vi "BuildThermomechanicalStave.vi"() -> ()   [LabVIEW 2016]
doc: "This VI is the overarching framework for the ITk Stave Assembly at Brookhaven National Lab. This VI coordinates all SubVIs so that the user can execute all phases of construction: Calibration, Module Placement, and Final Survey."
uses:
  <vilib>/userdefined/High Color/IMAQdx.ctl
  C:/Users/sciollalab/Documents/Brandeis-BNL/LabVIEW_Codes/BNL_ThermomechanicalStave/AerotechLibraries/Bin/Aerotech.A3200.dll
  AerotechLibraries/Bin/Aerotech.A3200.dll
  <vilib>/Utility/file.llb/Write Delimited Spreadsheet (DBL).vi
  <vilib>/vision/driver/NI_Vision_Acquisition_Software.lvlib
panel:
  out "Current time and temperature":string[](array[string])
  out "Wait to capture [ms]":u32
  in  "Wait time [s]":dbl=3.5
  in  "N pix/um images":i32=1
  out "Inputs: Collect images":T2={"Session in"="", "Axes Speeds [mm/s]"={"X Speed"=10.0, "Y Speed"=10.0, "Z Speed"=10.0}, "XYZ .NET Refnum in"=refnum, "Current image"=refnum, "Stage position"=refnum, "Moving"=refnum}
  out "XYZ Stage Control":refnum<k24>
  out "Baseline Z [mm]":dbl
  in  "Placement tolerance [um]":dbl=10.0
  out "Module Progress Report":T3(array[cluster])
  out "Surveyed?":bool
  out "Mounted?":bool
  out "Calibrated?":bool
  in  "N Modules":i32=13
  out "Calibrated module height":dbl
  out "Calibrated stave basis [mm]":dbl[][](array[numeric])
  out "Module fiducials in the XYZ stage's basis":T4(graph)=[{"Generated List of Module Coordinates"=[0.0, 280.05, 574.05, 868.05, 1162.05], "Generated List of Module Coordinates"=[0.0, 0.0, 0.0, 0.0, 0.0]}, {"Generated List of Module Coordinates"=[-7.689999999999998, 87.79, 87.79, -7.689999999999998, 90.31, 185.79000000000002, 185.79000000000002, 90.31, 188.31, 283.79, 283.79, 188.31, 286.31, 381.79, 381.79, 286.31, 384.31, 479.79, 479.79, 384.31, 482.30999999999995, 577.79, 577.79, 482.30999999999995, 580.31, 675.79, 675.79, 580.31, 678.31, 773.79, 773.79, 678.31, 776.31, 871.79, 871.79, 776.31, 874.31, 969.79, 969.79, 874.31, 972.31, 1067.79, 1067.79, 972.31, 1070.31, 1165.79, 1165.79, 1070.31, 1168.31, 1263.79, 1263.79, 1168.31], "Generated List of Module Coordinates"=[-113.212, -113.212, -16.13199999999999, -16.13199999999999, -113.212, -113.212, -16.13199999999999, -16.13199999999999, -113.212, -113.212, -16.13199999999999, -16.13199999999999, -113.212, -113.212, -16.13199999999999, -16.13199999999999, -113.212, -113.212, -16.13199999999999, -16.13199999999999, -113.212, -113.212, -16.13199999999999, -16.13199999999999, -113.212, -113.212, -16.13199999999999, -16.13199999999999, -113.212, -113.212, -16.13199999999999, -16.13199999999999, -113.212, -113.212, -16.13199999999999, -16.13199999999999, -113.212, -113.212, -16.13199999999999, -16.13199999999999, -113.212, -113.212, -16.13199999999999, -16.13199999999999, -113.212, -113.212, -16.13199999999999, -16.13199999999999, -113.212, -113.212, -16.13199999999999, -16.13199999999999]}, {"Generated List of Module Coordinates"=[40.050000000000004, 138.05, 236.05, 334.05, 432.05, 530.05, 628.05, 726.05, 824.05, 922.05, 1020.05, 1118.05, 1216.05], "Generated List of Module Coordinates"=[-64.672, -64.672, -64.672, -64.672, -64.672, -64.672, -64.672, -64.672, -64.672, -64.672, -64.672, -64.672, -64.672]}]
  in  "Home stage?":bool
  out "Calib Pattern":T5
  out "Autofocus":T5
  out "Stave origin":T5
  in  "XYZ Stage Frame: Coordinates for calibration":T6={"Stave origin"={"X [mm]"=-628.0, "Y [mm]"=142.3, "Z [mm]"=22.0}, "Autofocus"={"X [mm]"=-597.0, "Y [mm]"=132.0, "Z [mm]"=18.0}, "Calib Pattern"={"X [mm]"=-560.0, "Y [mm]"=112.0, "Z [mm]"=13.9}}
  out "Focusing test interval [mm]":dbl
  out "Stepsize [mm]":dbl
  in  "Camera working distance scan":T7={"Stepsize [mm]"=0.2, "Focusing test interval [mm]"=1.5} {"Focusing test interval [mm]" format="%#_13g"}
  out "Calibration Results":T8 {"Camera calibration results"."Working distance to stave [mm]" format="%#_13g"}
  out "delta Z":dbl
  in  "Reports path":path=path "C:/Users/Aerotech/cernbox/BNL/Stave Assembly Records/2017-04-05"
  in  "Code path":path=path "C:/Users/Aerotech/Documents/BNL_ThermomechanicalStave"
  out "Calibrated stave origin (X,Y) [mm]":dbl[](array[numeric])
  in  "Tape Type":enum16{"Stereo", "Axial"}(ring)=enum."Axial"
  out "Angle between stave and xyz stage":dbl
  in  "Module fiducial marker":T9(ring)=enum."Mark B"
  out "Average microns/pixel":ext
  out "Optimized Z [mm]":dbl format="%#_13g"
  out "Session Out":T1="cam0"
  out "Current stage position [mm]":cluster{"X":dbl, "Y":dbl, "Z":dbl}
  out "Moving":bool
  out "Stage homed":bool
  in  "Axis Speeds":T10={"X [mm/s]"=10.0, "Y [mm/s]"=10.0, "Z [mm/s]"=10.0}
  out "Current field of view":T11(plugin-control)
  in  "Camera Name":refnum<k21>="cam1" caption="IMAQdx Session"
  in  "Program Errors":errorcluster
  out "Current Build Phase":string="Going to nominal stave origin..."
  # "BUILD THERMOMECHANICAL STAVE"
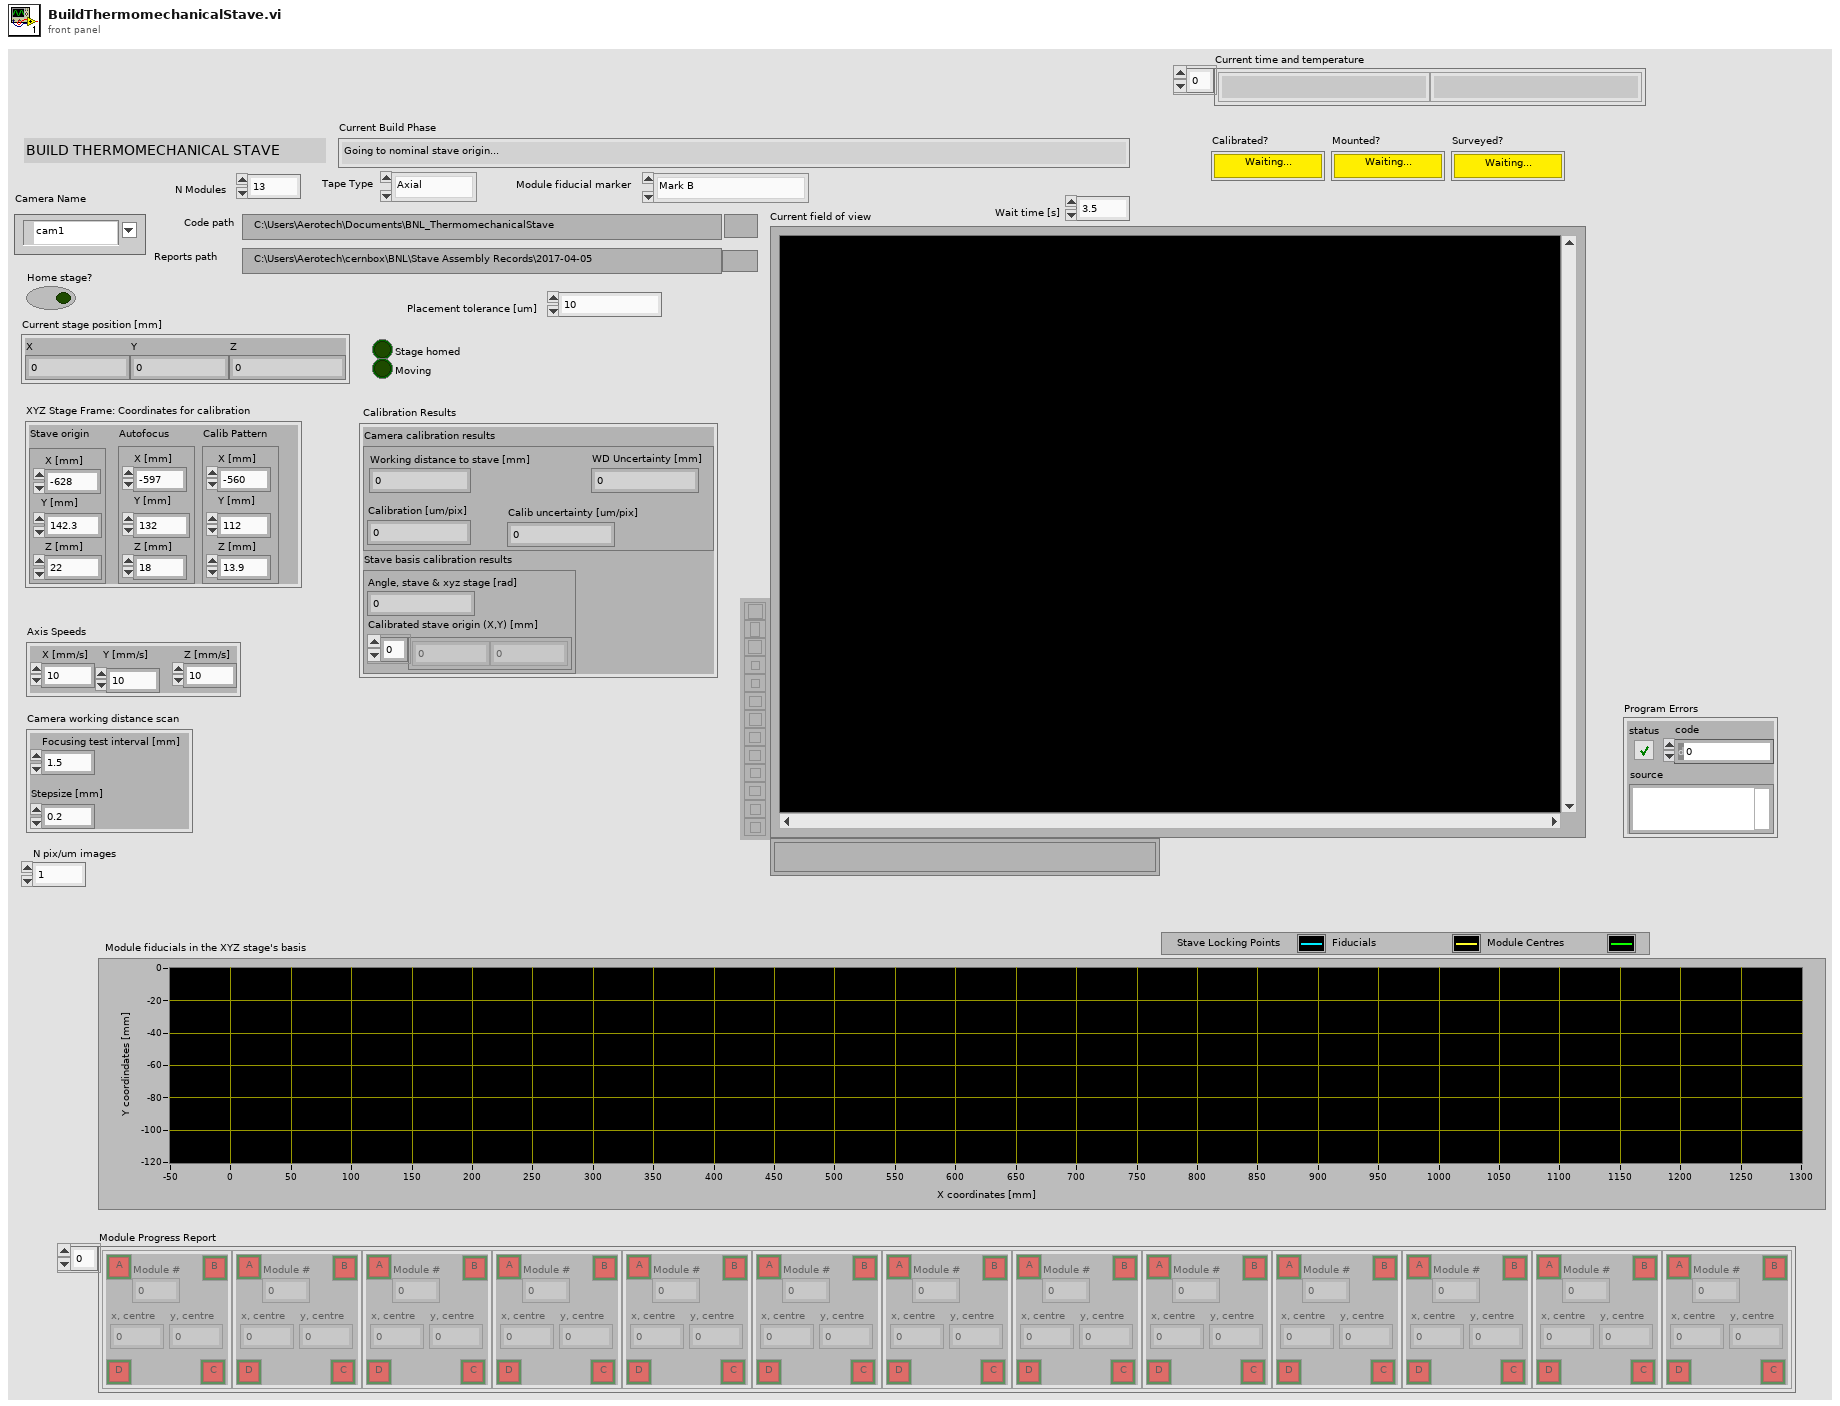
[diagram p1: front panel]
types:
  T1 = typedef "IMAQdx.ctl" = refnum<k21>
  T2 = cluster{"Session in":T1, "Axes Speeds [mm/s]":cluster{"X Speed":dbl, "Y Speed":dbl, "Z Speed":dbl}, "XYZ .NET Refnum in":refnum<k24>, "Current image":refnum<vi>, "Stage position":refnum<vi>, "Moving":refnum<vi>}
  T3 = cluster{"A":bool, "x, centre":dbl, "y, centre":dbl, "Module #":i32, "B":bool, "D":bool, "C":bool}[]
  T4 = cluster{"Generated List of Module Coordinates":dbl[], "Generated List of Module Coordinates":dbl[]}[]
  T5 = cluster{"X [mm]":dbl, "Y [mm]":dbl, "Z [mm]":dbl}
  T6 = cluster{"Stave origin":cluster{"X [mm]":dbl, "Y [mm]":dbl, "Z [mm]":dbl}, "Autofocus":cluster{"X [mm]":dbl, "Y [mm]":dbl, "Z [mm]":dbl}, "Calib Pattern":cluster{"X [mm]":dbl, "Y [mm]":dbl, "Z [mm]":dbl}}
  T7 = cluster{"Stepsize [mm]":dbl, "Focusing test interval [mm]":dbl}
  T8 = cluster{"Camera calibration results":cluster{"Calibration [um/pix]":dbl, "Working distance to stave [mm]":dbl, "Calib uncertainty [um/pix]":dbl, "WD Uncertainty [mm]":dbl}, "Stave basis calibration results":cluster{"Angle, stave & xyz stage [rad]":dbl, "Calibrated stave origin (X,Y) [mm]":dbl[]}}
  T9 = enum16{"Mark C", "Mark B", "Strip Corner", "[None]"}
  T10 = cluster{"X [mm/s]":dbl, "Y [mm/s]":dbl, "Z [mm/s]":dbl}
  T11 = typedef "IMAQ Image.ctl" = refnum<image>
  T12 = cluster{"X Position Feedback":dbl, "Y Position Feedback":dbl, "Z Position Feedback":dbl}
  T13 = cluster{"Final X":dbl, "Final Y":dbl, "Final Z":dbl}
  T14 = typedef "Image Type" = u32
  T15 = cluster{"Update X [mm]":dbl, "Update Y [mm]":dbl, "Update Z [mm]":dbl}
  T16 = cluster{"Update X [mm]":dbl, "Update Y [mm]":dbl, "Z [mm]":dbl}
  T17 = cluster{"Camera session out":T1, "Axis Speeds":cluster{"X [mm/s]":dbl, "Y [mm/s]":dbl, "Z [mm/s]":dbl}, "XYZ Stage Control":refnum<k24>, "Current field of view":refnum<vi>, "Current stage position [mm]":refnum<vi>, "Moving":refnum<vi>}
  T18 = cluster{"Session out":T1, "Captured positions":dbl[][], "XYZ .NET Refnum out":refnum<k24>}
  T19 = cluster{"Calibrated stave basis [mm]":dbl[], "Calibrated stave basis [mm]":dbl[]}
  T20 = cluster{"Calibrated stave basis [mm]":dbl[], "Calibrated stave basis [mm]":dbl[]}[]
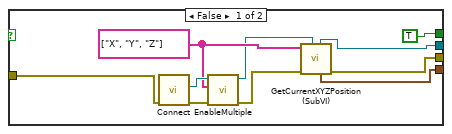
[diagram p2: hidden frame]
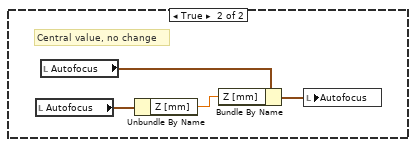
[diagram p13: hidden frame]
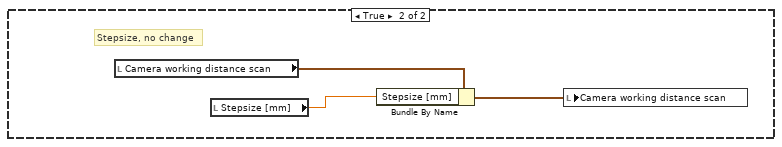
[diagram p14: hidden frame]
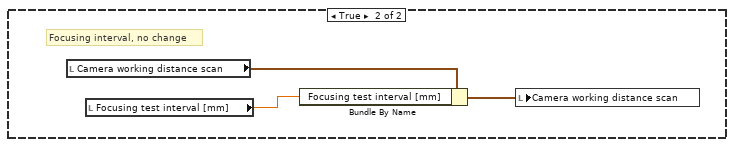
[diagram p15: hidden frame]
diagram:
  n1 = while {
    stop <- w17 stop-if-true
    # "Temperature monitoring"
    n2 = Wait (ms)(milliseconds to wait=u32 1000) -> ()  [unwired: 1 out]
    n3 = call "TimeAndTemperature (SubVI).vi"("Command"="FETC?", "GPIB Address: Temperature"="16") -> ("str( Time, Temp )"=→"Current time and temperature":string[])  [unwired: 6 in, 3 out]
    n4 = Multiply(x="Wait time [s]", y=u32 1000) -> (x*y=→"Wait to capture [ms]":dbl)
    n5 = local read "Surveyed?"() -> (w17:bool)
  }
  n6 = flat-sequence {
    tunnel: [w34] -> w8
    tunnel: [w24] -> w5
    tunnel: w8 -> [w61]
    tunnel: [w59] -> w7
    tunnel: w5 -> [w57]
    tunnel: w7 -> [w78]
    tunnel: [w75] -> w11
    tunnel: w11 -> [w492]
    tunnel: [w483] -> w2
    tunnel: [w538] -> w10
    tunnel: [w534] -> w3
    tunnel: w2 -> [w534]
    tunnel: w10 -> [w544]
    tunnel: [w543] -> w9
    tunnel: [w542] -> w4
    tunnel: w3 -> [w542]
    tunnel: w9 -> [w577]
    tunnel: [w577] -> w6
    tunnel: w4 -> [w572]
    tunnel: [w570] -> w1
    tunnel: w6 -> [w623]
    tunnel: w1 -> [w608]
    frame #0 {
      w21 = FALSE ("Stage homed")
      "Current Build Phase" <- "" ("Current Build Phase")
      "Moving" <- w21
      "Stage homed" <- w21
      "Calibration Results" <- T8 {"Camera calibration results"={"Calibration [um/pix]"=0.0, "Working distance to stave [mm]"=0.0, "Calib uncertainty [um/pix]"=0.0, "WD Uncertainty [mm]"=0.0}, "Stave basis calibration results"={"Angle, stave & xyz stage [rad]"=0.0, "Calibrated stave origin (X,Y) [mm]"=[0.0, 0.0]}} ("Calibration Results")
      "Surveyed?" <- w21
      "Calibrated?" <- w21
      "Mounted?" <- w21
      "Module Progress Report" <- T3 [] ("Module Progress Report")
    }
    frame #1 {
      # "Home the XYZ stage to activate its auto-calibration"
      n7 = property on="Calibration Results" class="Clust (strict)"() -> ("Controls[]"=w27:refnum<vi>[])  [unwired: 2 in, 2 out]
      n8 = local read "Program Errors"() -> (w29:errorcluster)
      n9 = local write "Moving"(TRUE ("Moving")) -> ()
      n10 = call "ConfigureLights (SubVI).vi"() -> ()  [unwired: 12 in]
      n11 = case shown="True" "Home stage?" {
        tunnel: [w39 w53] -> w37
        tunnel: [w47 w52] -> w34
        tunnel: w29 -> [w48 w51]
        tunnel: [TRUE ("completed") w50] -> w25
        tunnel: [w41 w49] -> w24
        frame False {
          w43 = string[] ["X", "Y", "Z"] ("Axes Names")
          n12 = call "Connect.vi"("error in (no error)"=w48) -> ("error out"=w45:errorcluster, "controller"=w44:refnum<k24>)  [unwired: 9 in]
          n13 = call "EnableMultiple.vi"("error in (no error)"=w45, "axis names"=w43, "controller in"=w44) -> ("error out"=w46:errorcluster, "controller out"=w42:refnum<k24>)  [unwired: 7 in]
          n14 = call "GetCurrentXYZPosition (SubVI).vi"(".NET Refnum in - Device"=w42, "error in (no error)"=w46, "Axes Names"=w43) -> ("error out"=w47:errorcluster, "Current stage position"=w39:T5, ".NET Refnum out  - Device"=w41:refnum<k24>)  [unwired: 3 in, 3 out]
        }
        frame True {
          n15 = call "0_HomeAllAxes (SubVI).vi"("error in (no error)"=w51) -> ("error out"=w52:errorcluster, "Homed coordinates"=w53:T12, "controller out"=w49:refnum<k24>, "completed"=w50:bool)  [unwired: 7 in]
        }
      }
      "Current stage position [mm]" <- w37
      "XYZ Stage Control" <- w24
      n16 = Index Array(array=w27, index=0) -> ()  [unwired: 1 out]
      n17 = local write "Current Build Phase"("Homing XYZ stage..." ("Current Build Phase")) -> ()
      n18 = Unbundle By Name("XYZ Stage Frame: Coordinates for calibration") -> ("Stave origin"=→"Stave origin":T5, "Autofocus"=→"Autofocus":T5, "Calib Pattern"=→"Calib Pattern":T5)
      n19 = Not(x=w25) -> (.not. x?=w36:bool)
      n20 = local write "Stage homed"(w25) -> ()
      n21 = local write "Moving"(w36) -> ()
    }
    frame #2 {
      n22 = local read "Axis Speeds"() -> (w55:T10)
      n23 = local read "Stave origin"() -> (w58:T5)
      n24 = local write "Moving"(TRUE ("Moving")) -> ()
      n25 = call "LightSwitch (SubVI).vi"("Spotlight"=TRUE) -> ()  [unwired: 11 in]
      n26 = call "Go2XYZ (SubVI).vi"(".NET Refnum in"=w57, "Go to Coordinates"=w58, "Axis Speeds"=w55, "error in (no error)"=w61) -> ("completed"=w63:bool, ".NET Refnum out"=w56:refnum<k24>, "Final Position"=w60:T13, "error out"=w59:errorcluster)  [unwired: 7 in, 1 out]
      n27 = Not(x=w63) -> (.not. x?=w64:bool)
      n28 = local write "XYZ Stage Control"(w56) -> ()
      n29 = local write "Current stage position [mm]"(w60) -> ()
      n30 = local write "Moving"(w64) -> ()
      n31 = local write "Current Build Phase"("Going to nominal stave origin..." ("Current Build Phase")) -> ()
    }
    frame #3 {
      w85 = T14 0 items=["Grayscale (U8)", "Grayscale (I16)", "Grayscale (SGL)", "Complex (CSG)", "RGB (U32)", "HSL (U32)", "RGB (U64)", "Grayscale (U16)"] ("Image Type")
      # "Connect to the camera VISA"
      n32 = call <vilib>:"IMAQdx Open Camera.vi"("error in"=w78, "Session In"="Camera Name") -> ("error out"=w83:errorcluster, "Session Out"=w82:T1)  [unwired: 1 in, 7 out]
      n33 = local write "Current Build Phase"("Connecting camera..." ("Current Build Phase")) -> ()
      n34 = call "IMAQ Create"("Image Name"="Grab", "Image Type"=w85, "error in (no error)"=w78) -> ("New Image"=w76:T11, "error out"=w77:errorcluster)  [unwired: 1 in, 1 out]
      n35 = call <vilib>:"IMAQdx Configure Grab.vi"("error in"=w83, "Session In"=w82) -> ("error out"=w79:errorcluster, "Session Out"=w80:T1)  [unwired: 8 out]
      n36 = flat-sequence {
        tunnel: w76 -> [w100]
        tunnel: w77 -> [w93]
        tunnel: w79 -> [w94]
        tunnel: w80 -> [w101]
        tunnel: [w92] -> w74
        tunnel: w74 -> [w105]
        tunnel: [w104] -> w69
        tunnel: [w173] -> w68
        tunnel: w69 -> [w174]
        tunnel: w68 -> [w242]
        tunnel: [w242] -> w67
        tunnel: w67 -> [w244]
        tunnel: [w243] -> w71
        tunnel: w71 -> [w314]
        tunnel: [w313] -> w70
        tunnel: [w428] -> w73
        tunnel: [w427] -> w72
        tunnel: w70 -> [w425]
        tunnel: w73 -> [w465]
        tunnel: w72 -> [w464]
        tunnel: [w473] -> w66
        tunnel: [w482] -> w75
        tunnel: w66 -> [w482]
        frame #0 {
          # "Configure the camera. When configuration\ncomplete, press \"Set cam settings\" to accept\nthem."
          n37 = Merge Errors(w93, w94) -> (w102:errorcluster)
          n38 = local read "Autofocus"() -> (w98:T5)
          n39 = call "0_SetupCameraAttributes (SubVI).vi"("error in (no error)"=w102, "Gain"=16.0 ("Camera gain"), "Camera session in"=w101) -> ("error out"=w96:errorcluster, "Camera session out"=w97:T1)  [unwired: 7 in]
          n40 = Unbundle By Name(w98) -> ("Z [mm]"=→"Baseline Z [mm]":dbl)
          n41 = call <vilib>:"IMAQdx Grab.vi"("error in"=w96, "Image In"=w100, "Session In"=w97) -> ("error out"=w87:errorcluster, "Image Out"=w90:T11, "Session Out"=w89:T1)  [unwired: 1 in, 5 out]
          n42 = call "AlignCameraFrame (SubVI).vi"("error in (no error)"=w87, "Image Src"=w90, "Camera session in"=w89) -> ("error out"=w92:errorcluster, "Image Dst Out"=→"Current field of view":T11, "Camera session out"=→"Session Out":T1)  [unwired: 6 in]
          n43 = local write "Current Build Phase"("Configuring camera..." ("Current Build Phase")) -> ()
        }
        frame #1 {
          n44 = while {
            tunnel: w105 -> [w119]
            tunnel: [w106] -> w104
            stop <- w118 stop-if-true
            n45 = flat-sequence {
              tunnel: w119 -> [w132]
              tunnel: [w125] -> w115
              tunnel: [w124] -> w113
              tunnel: [w123] -> w111
              tunnel: [w121] -> w108
              tunnel: w115 -> [w137]
              tunnel: [w137] -> w114
              tunnel: w113 -> [w136]
              tunnel: [w136] -> w112
              tunnel: w111 -> [w135]
              tunnel: [w135] -> w110
              tunnel: [w134] -> w109
              tunnel: w108 -> [w134]
              tunnel: w114 -> [w155]
              tunnel: w112 -> [w147]
              tunnel: w110 -> [w146]
              tunnel: [w158] -> w117
              tunnel: [w145] -> w116
              tunnel: w109 -> [w140]
              tunnel: [w138] -> w107
              tunnel: [w166] -> w118
              tunnel: w117 -> [w165]
              tunnel: w116 -> [w170]
              tunnel: w107 -> [w169]
              tunnel: [w168] -> w106
              frame #0 {
                n46 = local read "XYZ Stage Control"() -> (w128:refnum<k24>)
                n47 = local read "Stave origin"() -> (w122:T5)
                n48 = local read "Axis Speeds"() -> (w126:T10)
                n49 = Unbundle By Name(w122) -> ("X [mm]"=w125:dbl, "Y [mm]"=w124:dbl, "Z [mm]"=w123:dbl)
                n50 = call "Go2XYZ (SubVI).vi"(".NET Refnum in"=w128, "Go to Coordinates"=w122, "Axis Speeds"=w126, "error in (no error)"=w132) -> ("completed"=w130:bool, ".NET Refnum out"=w127:refnum<k24>, "Final Position"=w129:T13, "error out"=w121:errorcluster)  [unwired: 7 in, 1 out]
                n51 = Not(x=w130) -> (.not. x?=w131:bool)
                n52 = local write "XYZ Stage Control"(w127) -> ()
                n53 = local write "Current stage position [mm]"(w129) -> ()
                n54 = local write "Moving"(w131) -> ()
              }
              frame #1 {
                n55 = local read "Wait to capture [ms]"() -> (w133:u32)
                n56 = Wait (ms)(milliseconds to wait=w133) -> ()  [unwired: 1 out]
              }
              frame #2 {
                n57 = local read "Current field of view"() -> (w141:T11)
                n58 = local read "Session Out"() -> (w142:T1)
                n59 = call <vilib>:"IMAQdx Grab.vi"("error in"=w140, "Image In"=w141, "Session In"=w142) -> ("error out"=w139:errorcluster, "Image Out"=w144:T11, "Session Out"=w143:T1)  [unwired: 1 in, 5 out]
                n60 = call "Accept nominal stave origin"("error in (no error)"=w139) -> ("Update Z [mm]"=w149:dbl, "Update Y [mm]"=w151:dbl, "Update X [mm]"=w156:dbl, "Accept stave origin"=w158:bool, "error out"=w138:errorcluster)  [unwired: 13 in, 1 out]
                n61 = local write "Session Out"(w143) -> ()
                n62 = local write "Current field of view"(w144) -> ()
                n63 = Not Equal To 0?(x=w156) -> (x != 0?=w157:bool)
                n64 = Not Equal To 0?(x=w151) -> (x != 0?=w153:bool)
                n65 = Not Equal To 0?(x=w149) -> (x != 0?=w152:bool)
                n66 = case shown="False" w157 {
                  tunnel: [w163 w164] -> w154
                  tunnel: w156 -> [_ w164]
                  tunnel: w155 -> [w163 _]
                  frame False {
                  }
                  frame True {
                  }
                }
                n67 = case shown="False" w153 {
                  tunnel: w151 -> [_ w162]
                  tunnel: [w161 w162] -> w150
                  tunnel: w147 -> [w161 _]
                  frame False {
                  }
                  frame True {
                  }
                }
                n68 = case shown="False" w152 {
                  tunnel: w149 -> [_ w160]
                  tunnel: [w159 w160] -> w148
                  tunnel: w146 -> [w159 _]
                  frame False {
                  }
                  frame True {
                  }
                }
                n69 = Bundle("Update X [mm]"=w154, "Update Y [mm]"=w150, "Update Z [mm]"=w148) -> (w145:T15)  [unwired: 1 in]
                n70 = local write "Stave origin"(w145) -> ()
              }
              frame #3 {
                n71 = call <vilib>:"General Error Handler.vi"("error in (no error)"=w169) -> ("error?"=w167:bool, "error out"=w168:errorcluster)  [unwired: 10 in, 3 out]
                n72 = local read "XYZ Stage Frame: Coordinates for calibration"() -> (w172:T6)
                n73 = Or(x=w165, y=w167) -> (x .or. y?=w166:bool)
                n74 = Bundle By Name(cluster=w172, "Stave origin"=w170) -> (w171:T6)
                n75 = local write "XYZ Stage Frame: Coordinates for calibration"(w171) -> ()
              }
            }
            n76 = local write "Current Build Phase"("Check initial coordinates: Nominal origin..." ("Current Build Phase")) -> ()
          }
        }
        frame #2 {
          n77 = while {
            tunnel: w174 -> [w188]
            tunnel: [w175] -> w173
            stop <- w187 stop-if-true
            n78 = flat-sequence {
              tunnel: w188 -> [w201]
              tunnel: [w194] -> w184
              tunnel: [w193] -> w182
              tunnel: [w192] -> w180
              tunnel: [w190] -> w177
              tunnel: w184 -> [w206]
              tunnel: [w206] -> w183
              tunnel: w182 -> [w205]
              tunnel: [w205] -> w181
              tunnel: w180 -> [w204]
              tunnel: [w204] -> w179
              tunnel: [w203] -> w178
              tunnel: w177 -> [w203]
              tunnel: w183 -> [w224]
              tunnel: w181 -> [w216]
              tunnel: w179 -> [w215]
              tunnel: [w227] -> w186
              tunnel: [w214] -> w185
              tunnel: w178 -> [w209]
              tunnel: [w207] -> w176
              tunnel: [w235] -> w187
              tunnel: w186 -> [w236]
              tunnel: w185 -> [w239]
              tunnel: w176 -> [w238]
              tunnel: [w237] -> w175
              frame #0 {
                n79 = local read "XYZ Stage Control"() -> (w197:refnum<k24>)
                n80 = local read "Axis Speeds"() -> (w195:T10)
                n81 = local read "Autofocus"() -> (w191:T5)
                n82 = Unbundle By Name(w191) -> ("X [mm]"=w194:dbl, "Y [mm]"=w193:dbl, "Z [mm]"=w192:dbl)
                n83 = call "Go2XYZ (SubVI).vi"(".NET Refnum in"=w197, "Go to Coordinates"=w191, "Axis Speeds"=w195, "error in (no error)"=w201) -> ("completed"=w199:bool, ".NET Refnum out"=w196:refnum<k24>, "Final Position"=w198:T13, "error out"=w190:errorcluster)  [unwired: 7 in, 1 out]
                n84 = Not(x=w199) -> (.not. x?=w200:bool)
                n85 = local write "XYZ Stage Control"(w196) -> ()
                n86 = local write "Current stage position [mm]"(w198) -> ()
                n87 = local write "Moving"(w200) -> ()
              }
              frame #1 {
                n88 = local read "Wait to capture [ms]"() -> (w202:u32)
                n89 = Wait (ms)(milliseconds to wait=w202) -> ()  [unwired: 1 out]
              }
              frame #2 {
                n90 = local read "Current field of view"() -> (w210:T11)
                n91 = local read "Session Out"() -> (w211:T1)
                n92 = call <vilib>:"IMAQdx Grab.vi"("error in"=w209, "Image In"=w210, "Session In"=w211) -> ("error out"=w208:errorcluster, "Image Out"=w213:T11, "Session Out"=w212:T1)  [unwired: 1 in, 5 out]
                n93 = call "Accept autofocusing position"("error in (no error)"=w208) -> ("Update Z [mm]"=w218:dbl, "Update Y [mm]"=w220:dbl, "Update X [mm]"=w225:dbl, "Accept autofocusing position"=w227:bool, "error out"=w207:errorcluster)  [unwired: 13 in, 1 out]
                n94 = local write "Session Out"(w212) -> ()
                n95 = local write "Current field of view"(w213) -> ()
                n96 = Not Equal To 0?(x=w225) -> (x != 0?=w226:bool)
                n97 = Not Equal To 0?(x=w220) -> (x != 0?=w222:bool)
                n98 = Not Equal To 0?(x=w218) -> (x != 0?=w221:bool)
                n99 = case shown="False" w226 {
                  tunnel: [w232 w233] -> w223
                  tunnel: w225 -> [_ w233]
                  tunnel: w224 -> [w232 _]
                  frame False {
                  }
                  frame True {
                  }
                }
                n100 = case shown="False" w222 {
                  tunnel: w220 -> [_ w231]
                  tunnel: [w230 w231] -> w219
                  tunnel: w216 -> [w230 _]
                  frame False {
                  }
                  frame True {
                  }
                }
                n101 = case shown="False" w221 {
                  tunnel: w218 -> [_ w229]
                  tunnel: [w228 w229] -> w217
                  tunnel: w215 -> [w228 _]
                  frame False {
                  }
                  frame True {
                  }
                }
                n102 = Bundle("Update X [mm]"=w223, "Update Y [mm]"=w219, "Update Z [mm]"=w217) -> (w214:T15)  [unwired: 1 in]
                n103 = local write "Autofocus"(w214) -> ()
              }
              frame #3 {
                n104 = call <vilib>:"General Error Handler.vi"("error in (no error)"=w238) -> ("error?"=w234:bool, "error out"=w237:errorcluster)  [unwired: 10 in, 3 out]
                n105 = local read "XYZ Stage Frame: Coordinates for calibration"() -> (w241:T6)
                n106 = Or(x=w236, y=w234) -> (x .or. y?=w235:bool)
                n107 = Bundle By Name(cluster=w241, "Autofocus"=w239) -> (w240:T6)
                n108 = local write "XYZ Stage Frame: Coordinates for calibration"(w240) -> ()
              }
            }
            n109 = local write "Current Build Phase"("Check initial coordinates: autofocusing..." ("Current Build Phase")) -> ()
          }
        }
        frame #3 {
          n110 = call "LightSwitch (SubVI).vi"() -> ()  [unwired: 12 in]
        }
        frame #4 {
          n111 = while {
            tunnel: [w247] -> w243
            tunnel: w244 -> [w251]
            stop <- w248 stop-if-true
            n112 = flat-sequence {
              tunnel: [w268] -> w259
              tunnel: [w267] -> w257
              tunnel: [w266] -> w255
              tunnel: [w264] -> w252
              tunnel: w251 -> [w263]
              tunnel: w259 -> [w283]
              tunnel: [w283] -> w258
              tunnel: w257 -> [w282]
              tunnel: [w282] -> w256
              tunnel: w255 -> [w281]
              tunnel: [w281] -> w254
              tunnel: [w278] -> w253
              tunnel: w252 -> [w279]
              tunnel: [w277] -> w245
              tunnel: w258 -> [w298]
              tunnel: w256 -> [w293]
              tunnel: w254 -> [w286]
              tunnel: [w301] -> w261
              tunnel: [w292] -> w260
              tunnel: w253 -> [w288]
              tunnel: [w285] -> w246
              tunnel: w245 -> [w284]
              tunnel: w261 -> [w309]
              tunnel: w260 -> [w310]
              tunnel: [w309] -> w250
              tunnel: [w308] -> w249
              tunnel: [w307] -> w247
              tunnel: w246 -> [w306]
              frame #0 {
                n113 = local read "XYZ Stage Control"() -> (w271:refnum<k24>)
                n114 = local read "Calib Pattern"() -> (w265:T5)
                n115 = local read "Axis Speeds"() -> (w269:T10)
                n116 = Unbundle By Name(w265) -> ("X [mm]"=w268:dbl, "Y [mm]"=w267:dbl, "Z [mm]"=w266:dbl)
                n117 = call "Go2XYZ (SubVI).vi"(".NET Refnum in"=w271, "Go to Coordinates"=w265, "Axis Speeds"=w269, "error in (no error)"=w263) -> ("completed"=w273:bool, ".NET Refnum out"=w270:refnum<k24>, "Final Position"=w272:T13, "error out"=w264:errorcluster)  [unwired: 7 in, 1 out]
                n118 = Not(x=w273) -> (.not. x?=w274:bool)
                n119 = local write "XYZ Stage Control"(w270) -> ()
                n120 = local write "Current stage position [mm]"(w272) -> ()
                n121 = local write "Moving"(w274) -> ()
              }
              frame #1 {
                n122 = local read "Session Out"() -> (w276:T1)
                n123 = local read "Wait to capture [ms]"() -> (w280:u32)
                n124 = call "0_SetupCameraAttributes (SubVI).vi"("error in (no error)"=w279, "Gain"=0.0, "Camera session in"=w276) -> ("error out"=w278:errorcluster, "Camera session out"=w277:T1)  [unwired: 7 in]
                n125 = Wait (ms)(milliseconds to wait=w280) -> ()  [unwired: 1 out]
              }
              frame #2 {
                n126 = local read "Current field of view"() -> (w289:T11)
                n127 = call <vilib>:"IMAQdx Grab.vi"("error in"=w288, "Image In"=w289, "Session In"=w284) -> ("error out"=w287:errorcluster, "Image Out"=w291:T11, "Session Out"=w290:T1)  [unwired: 1 in, 5 out]
                n128 = call "Accept calibration pattern position"("error in (no error)"=w287) -> ("Update Y [mm]"=w295:dbl, "Update X [mm]"=w299:dbl, "Accept calibration pattern position"=w301:bool, "error out"=w285:errorcluster)  [unwired: 13 in, 2 out]
                n129 = local write "Session Out"(w290) -> ()
                n130 = local write "Current field of view"(w291) -> ()
                n131 = Not Equal To 0?(x=w299) -> (x != 0?=w300:bool)
                n132 = Not Equal To 0?(x=w295) -> (x != 0?=w296:bool)
                n133 = case shown="False" w300 {
                  tunnel: [w304 w305] -> w297
                  tunnel: w299 -> [_ w305]
                  tunnel: w298 -> [w304 _]
                  frame False {
                  }
                  frame True {
                  }
                }
                n134 = case shown="False" w296 {
                  tunnel: w295 -> [_ w303]
                  tunnel: [w302 w303] -> w294
                  tunnel: w293 -> [w302 _]
                  frame False {
                  }
                  frame True {
                  }
                }
                n135 = Bundle("Update X [mm]"=w297, "Update Y [mm]"=w294, "Z [mm]"=w286) -> (w292:T16)  [unwired: 1 in]
                n136 = local write "Calib Pattern"(w292) -> ()
              }
              frame #3 {
                n137 = local read "XYZ Stage Frame: Coordinates for calibration"() -> (w312:T6)
                n138 = Bundle By Name(cluster=w312, "Calib Pattern"=w310) -> (w311:T6)
                n139 = local write "XYZ Stage Frame: Coordinates for calibration"(w311) -> ()
                n140 = call <vilib>:"General Error Handler.vi"("error in (no error)"=w306) -> ("error?"=w308:bool, "error out"=w307:errorcluster)  [unwired: 10 in, 3 out]
              }
            }
            n141 = local write "Current Build Phase"("Check initial coordinates: calibration pattern..." ("Current Build Phase")) -> ()
            n142 = Or(x=w250, y=w249) -> (x .or. y?=w248:bool)
          }
        }
        frame #5 {
          n143 = while {
            tunnel: [w324] -> w313
            tunnel: w314 -> [w315]
            i -> [w322]
            stop <- w316 stop-if-true
            n144 = flat-sequence {
              tunnel: w322 -> [w342]
              tunnel: [w332] -> w321
              tunnel: [w331] -> w320
              tunnel: [w328] -> w319
              tunnel: w315 -> [w326]
              tunnel: [w387] -> w323
              tunnel: w321 -> [w369]
              tunnel: w320 -> [w380]
              tunnel: w319 -> [w379]
              tunnel: w323 -> [w395]
              tunnel: [w395] -> w318
              tunnel: [w394] -> w317
              tunnel: [w417] -> w324
              tunnel: w318 -> [w418]
              tunnel: w317 -> [w421]
              tunnel: [w420] -> w316
              frame #0 {
                n145 = local read "Reports path"() -> (w327:path)
                n146 = Build Path(base path=w327, name or relative path="autofocusing") -> (appended path=w345:path)
                n147 = call <vilib>:"Check if File or Folder Exists.vi"("error in (no error)"=w326, "path"=w345) -> ("error out"=w338:errorcluster, "file or folder exists?"=w341:bool, "dup path"=w339:path)  [unwired: 7 in]
                n148 = case shown="False" w341 {
                  tunnel: [w358 w359] -> w333
                  tunnel: [w357 w360] -> w329
                  tunnel: w339 -> [w355 w360]
                  tunnel: w338 -> [w356 w359]
                  frame False {
                    n149 = Create Folder(path (use dialog)=w355, error in=w356) -> (created path=w357:path, error out=w358:errorcluster)  [unwired: 1 in, 1 out]
                  }
                  frame True {
                  }
                }
                n150 = Unbundle By Name("Camera working distance scan") -> ("Stepsize [mm]"=→"Stepsize [mm]":dbl, "Focusing test interval [mm]"=→"Focusing test interval [mm]":dbl)
                n151 = call "LightSwitch (SubVI).vi"("Spotlight"=TRUE) -> ()  [unwired: 11 in]
                n152 = Number To Decimal String(number=w342) -> (decimal integer string=w330:string)  [unwired: 1 in]
                n153 = Build Path(base path=w329, name or relative path=w330) -> (appended path=w334:path)
                n154 = call <vilib>:"Check if File or Folder Exists.vi"("error in (no error)"=w333, "path"=w334) -> ("error out"=w337:errorcluster, "file or folder exists?"=w335:bool, "dup path"=w336:path)  [unwired: 7 in]
                n155 = local read "Code path"() -> (w343:path)
                n156 = case shown="False" w335 {
                  tunnel: [w352 w353] -> w331
                  tunnel: [w351 w354] -> w332
                  tunnel: w336 -> [w350 w354]
                  tunnel: w337 -> [w349 w353]
                  frame False {
                    n157 = Create Folder(path (use dialog)=w350, error in=w349) -> (created path=w351:path, error out=w352:errorcluster)  [unwired: 1 in, 1 out]
                  }
                  frame True {
                  }
                }
                n158 = Build Path(base path=w343, name or relative path="0_Calibration") -> (appended path=w328:path)
              }
              frame #1 {
                n159 = local read "Session Out"() -> (w363:T1)
                n160 = control-ref of="Current stage position [mm]"() -> (w374:refnum<vi>)
                n161 = local read "XYZ Stage Control"() -> (w376:refnum<k24>)
                n162 = control-ref of="Current field of view"() -> (w375:refnum<vi>)
                n163 = local read "Focusing test interval [mm]"() -> (w385:dbl)
                n164 = local read "Axis Speeds"() -> (w377:T10)
                n165 = local read "Wait to capture [ms]"() -> (w364:u32)
                n166 = call "0_SetupCameraAttributes (SubVI).vi"("Gain"=16.0, "Camera session in"=w363) -> ("Camera session out"=w361:T1)  [unwired: 8 in, 1 out]
                n167 = control-ref of="Moving"() -> (w373:refnum<vi>)
                n168 = control-ref of="Current Build Phase"() -> (w372:refnum<vi>)
                n169 = local read "Stepsize [mm]"() -> (w384:dbl)
                n170 = local read "Autofocus"() -> (w378:T5)
                n171 = local read "Calibration Results"() -> (w383:T8)
                n172 = local read "Baseline Z [mm]"() -> (w381:dbl)
                n173 = Bundle("Camera session out"=w361, "Axis Speeds"=w377, "XYZ Stage Control"=w376, "Current field of view"=w375, "Current stage position [mm]"=w374, "Moving"=w373) -> (w368:T17)  [unwired: 1 in]
                "Inputs: Collect images" <- w368
                n174 = call "1_FindWorkingZDistance.vi"("Inputs: Collect Images"=w368, "Current Build Phase"=w372, "Autofocus Coordinates"=w378, "Focusing test range [mm]"=w385, "Stepsize [mm]"=w384, "error in (no error)"=w380, "Templates directory"=w379, "Path to save collected images"=w369, "milliseconds to wait"=w364) -> ("Optimized working distance"=w365:dbl, "Uncertainty on optimized Z"=w371:dbl, "Outputs: Collect Images"=w370:T18, "error out"=w387:errorcluster)  [unwired: 7 in]
                "Optimized Z [mm]" <- w365
                n175 = Bundle By Name(cluster=w383, "Camera calibration results.Working distance to stave [mm]"=w365, "Camera calibration results.WD Uncertainty [mm]"=w371) -> (w382:T8)
                n176 = Subtract(x=w381, y=w365) -> (x-y=→"delta Z":dbl)
                n177 = Unbundle By Name(w370) -> ("Session out"=w367:T1, "XYZ .NET Refnum out"=w366:refnum<k24>)
                n178 = local write "Session Out"(w367) -> ()
                n179 = local write "XYZ Stage Control"(w366) -> ()
                n180 = local write "Calibration Results"(w382) -> ()
              }
              frame #2 {
                n181 = call "Accept calculated working distance"() -> ("Update stepsize [mm]"=w391:dbl, "Update focusing interval [mm]"=w390:dbl, "Update central value [mm]"=w388:dbl, "Accept working distance"=w394:bool)  [unwired: 14 in, 2 out]
                n182 = Equal To 0?(x=w388) -> (x = 0?=w389:bool)
                n183 = Equal To 0?(x=w391) -> (x = 0?=w392:bool)
                n184 = Equal To 0?(x=w390) -> (x = 0?=w393:bool)
                n185 = case shown="False" w389 {
                  tunnel: w388 -> [w396 _]
                  frame False {
                    # "Focusing interval changes"
                    n186 = local read "Autofocus"() -> (w397:T5)
                    n187 = Bundle By Name(cluster=w397, "Z [mm]"=w396) -> (w398:T5)
                    n188 = local write "Autofocus"(w398) -> ()
                  }
                  frame True {
                    # "Central value, no change"
                    n189 = local read "Autofocus"() -> (w400:T5)
                    n190 = local read "Autofocus"() -> (w401:T5)
                    n191 = Unbundle By Name(w400) -> ("Z [mm]"=w399:dbl)
                    n192 = Bundle By Name(cluster=w401, "Z [mm]"=w399) -> (w402:T5)
                    n193 = local write "Autofocus"(w402) -> ()
                  }
                }
                n194 = case shown="False" w392 {
                  tunnel: w391 -> [w404 _]
                  tunnel: w391 -> [w403 _]
                  frame False {
                    # "Stepsize changes"
                    n195 = local write "Stepsize [mm]"(w403) -> ()
                    n196 = local read "Camera working distance scan"() -> (w405:T7)
                    n197 = Bundle By Name(cluster=w405, "Stepsize [mm]"=w404) -> (w406:T7)
                    n198 = local write "Camera working distance scan"(w406) -> ()
                  }
                  frame True {
                    # "Stepsize, no change"
                    n199 = local read "Camera working distance scan"() -> (w408:T7)
                    n200 = local read "Stepsize [mm]"() -> (w407:dbl)
                    n201 = Bundle By Name(cluster=w408, "Stepsize [mm]"=w407) -> (w409:T7)
                    n202 = local write "Camera working distance scan"(w409) -> ()
                  }
                }
                n203 = case shown="False" w393 {
                  tunnel: w390 -> [w411 _]
                  tunnel: w390 -> [w410 _]
                  frame False {
                    # "Focusing interval changes"
                    n204 = local write "Focusing test interval [mm]"(w410) -> ()
                    n205 = local read "Camera working distance scan"() -> (w412:T7)
                    n206 = Bundle By Name(cluster=w412, "Focusing test interval [mm]"=w411) -> (w413:T7)
                    n207 = local write "Camera working distance scan"(w413) -> ()
                  }
                  frame True {
                    # "Focusing interval, no change"
                    n208 = local read "Camera working distance scan"() -> (w415:T7)
                    n209 = local read "Focusing test interval [mm]"() -> (w414:dbl)
                    n210 = Bundle By Name(cluster=w415, "Focusing test interval [mm]"=w414) -> (w416:T7)
                    n211 = local write "Camera working distance scan"(w416) -> ()
                  }
                }
              }
              frame #3 {
                n212 = call <vilib>:"General Error Handler.vi"("error in (no error)"=w418) -> ("error?"=w419:bool, "error out"=w417:errorcluster)  [unwired: 10 in, 3 out]
                n213 = local read "XYZ Stage Frame: Coordinates for calibration"() -> (w424:T6)
                n214 = Or(x=w419, y=w421) -> (x .or. y?=w420:bool)
                n215 = local read "Autofocus"() -> (w422:T5)
                n216 = Bundle By Name(cluster=w424, "Autofocus"=w422) -> (w423:T6)
                n217 = local write "XYZ Stage Frame: Coordinates for calibration"(w423) -> ()
              }
            }
          }
        }
        frame #6 {
          # "- Determine the appropriate height for the \ncamera above the sample\n- Return change in pixels per length as a function\nof height"
          n218 = call "LightSwitch (SubVI).vi"() -> ()  [unwired: 12 in]
          n219 = local read "Calib Pattern"() -> (w439:T5)
          n220 = Unbundle By Name(w439) -> ("X [mm]"=w444:dbl, "Y [mm]"=w445:dbl, "Z [mm]"=w438:dbl)
          n221 = local read "delta Z"() -> (w447:dbl)
          n222 = local read "Inputs: Collect images"() -> (w433:T2)
          n223 = local read "Reports path"() -> (w453:path)
          n224 = local read "Session Out"() -> (w435:T1)
          n225 = Add(x=w438, y=w447) -> (x+y=w446:dbl)
          "Calibrated module height" <- w446
          n226 = Bundle By Name(cluster=w439, "X [mm]"=w444, "Y [mm]"=w445, "Z [mm]"=w446) -> (w441:T5)
          n227 = local write "Current Build Phase"("Finding calibration pattern..." ("Current Build Phase")) -> ()
          n228 = Build Path(base path=w453, name or relative path="pix_um_calib") -> (appended path=w450:path)
          n229 = call "0_SetupCameraAttributes (SubVI).vi"("error in (no error)"=w425, "Gain"=0.0 ("y"), "Camera session in"=w435) -> ("error out"=w443:errorcluster, "Camera session out"=w434:T1)  [unwired: 7 in]
          n230 = local read "XYZ Stage Control"() -> (w436:refnum<k24>)
          n231 = Cluster To Array(cluster=w441) -> (array=w440:dbl[])
          n232 = call <vilib>:"Check if File or Folder Exists.vi"("error in (no error)"=w443, "path"=w450) -> ("error out"=w449:errorcluster, "file or folder exists?"=w451:bool)  [unwired: 7 in, 1 out]
          n233 = for {
            N: "N pix/um images" -> [_]
            tunnel: w440 -> [w462]
            tunnel: [w462] -> w437 mode=indexing
          }
          n234 = case shown="False" w451 {
            tunnel: w450 -> [w459 w461]
            tunnel: [w458 w461] -> w427
            tunnel: w449 -> [w457 w460]
            tunnel: [w456 w460] -> w448
            frame False {
              n235 = Create Folder(path (use dialog)=w459, error in=w457) -> (created path=w458:path, error out=w456:errorcluster)  [unwired: 1 in, 1 out]
            }
            frame True {
            }
          }
          n236 = Bundle By Name(cluster=w433, "Session in"=w434, "XYZ .NET Refnum in"=w436) -> (w432:T2)
          n237 = local read "Wait to capture [ms]"() -> (w426:u32)
          n238 = call "CollectImageSet (SubVI).vi"("Inputs"=w432, "Path to save collected images"=w427, "milliseconds to wait"=w426, "Set of coordinates to process"=w437, "error in"=w448) -> ("Outputs"=w429:T18, "error out"=w428:errorcluster)  [unwired: 8 in, 1 out]
          n239 = Unbundle By Name(w429) -> ("Session out"=w431:T1, "XYZ .NET Refnum out"=w430:refnum<k24>)
          n240 = local write "Session Out"(w431) -> ()
          n241 = local write "XYZ Stage Control"(w430) -> ()
        }
        frame #7 {
          # "Determine the pixel to micron conversion"
          n242 = local read "Code path"() -> (w471:path)
          n243 = Build Path(base path=w471, name or relative path="0_Calibration") -> (appended path=w469:path)
          n244 = control-ref of="Current field of view"() -> (w468:refnum<vi>)
          n245 = local read "Calibration Results"() -> (w475:T8)
          n246 = Build Path(base path=w469, name or relative path="1_Camera") -> (appended path=w476:path)
          n247 = local write "Current Build Phase"("Calculating pixel-micron conversion..." ("Current Build Phase")) -> ()
          n248 = Build Path(base path=w476, name or relative path="2_10Strips_PixMicronCalibTemplate_10mpx.png") -> (appended path=w478:path)
          n249 = call "FetchImageSet (SubVI).vi"("error in (no error)"=w465, "Naming Convention"="*.png", "Images Directory"=w464) -> ("error out"=w466:errorcluster, "Image Array"=w467:T11[])  [unwired: 6 in, 1 out]
          n250 = call "2_PixelToMicronConversion (SubVI).vi"("Current image"=w468, "Template Image"=w478, "Images Array"=w467) -> ("Average microns/pixel"=w473:ext, "standard dev on microns/pixel"=w472:ext)  [unwired: 7 in]
          "Average microns/pixel" <- w473
          n251 = local write "Program Errors"(w466) -> ()
          n252 = Bundle By Name(cluster=w475, "Camera calibration results.Calibration [um/pix]"=w473, "Camera calibration results.Calib uncertainty [um/pix]"=w472) -> (w474:T8)
          n253 = local write "Calibration Results"(w474) -> ()
        }
        frame #8 {
          n254 = call "LightSwitch (SubVI).vi"("Spotlight"=TRUE) -> ()  [unwired: 11 in]
        }
      }
    }
    frame #4 {
      n255 = local read "Reports path"() -> (w519:path)
      n256 = local read "Program Errors"() -> (w514:errorcluster)
      n257 = local read "Stave origin"() -> (w498:T5)
      n258 = Build Path(base path=w519, name or relative path="staveCalib") -> (appended path=w516:path)
      n259 = call <vilib>:"Check if File or Folder Exists.vi"("error in (no error)"=w514, "path"=w516) -> ("error out"=w515:errorcluster, "file or folder exists?"=w517:bool)  [unwired: 7 in, 1 out]
      n260 = local read "Program Errors"() -> (w505:errorcluster)
      n261 = local read "Session Out"() -> (w507:T1)
      n262 = case shown="False" w517 {
        tunnel: w516 -> [w531 w533]
        tunnel: [w530 w533] -> w512
        tunnel: w515 -> [w529 w532]
        tunnel: [w528 w532] -> w513
        frame False {
          n263 = Create Folder(path (use dialog)=w531, error in=w529) -> (created path=w530:path, error out=w528:errorcluster)  [unwired: 1 in, 1 out]
        }
        frame True {
        }
      }
      n264 = Unbundle By Name(w498) -> ("X [mm]"=w508:dbl, "Y [mm]"=w509:dbl, "Z [mm]"=w500:dbl)
      n265 = local read "delta Z"() -> (w511:dbl)
      n266 = local write "Current Build Phase"("Locating locking points..." ("Current Build Phase")) -> ()
      n267 = local read "Code path"() -> (w496:path)
      n268 = control-ref of="Current stage position [mm]"() -> (w491:refnum<vi>)
      n269 = local read "Wait to capture [ms]"() -> (w484:u32)
      n270 = Add(x=w500, y=w511) -> (x+y=w510:dbl)
      n271 = local read "XYZ Stage Control"() -> (w487:refnum<k24>)
      n272 = control-ref of="Current Build Phase"() -> (w489:refnum<vi>)
      n273 = local read "Axis Speeds"() -> (w525:T10)
      n274 = control-ref of="Moving"() -> (w493:refnum<vi>)
      n275 = Bundle By Name(cluster=w498, "X [mm]"=w508, "Y [mm]"=w509, "Z [mm]"=w510) -> (w499:T5)
      n276 = Build Path(base path=w496, name or relative path="0_Calibration") -> (appended path=w494:path)
      n277 = call "0_SetupCameraAttributes (SubVI).vi"("error in (no error)"=w505, "Gain"=16.0, "Camera session in"=w507) -> ("error out"=w504:errorcluster, "Camera session out"=w506:T1)  [unwired: 7 in]
      n278 = control-ref of="Current field of view"() -> (w490:refnum<vi>)
      n279 = control-ref of="Calibration Results"() -> (w488:refnum<vi>)
      n280 = call "0_StageToStave.vi"("Cam session in"=w506, "Stave origin in XYZ Frame"=w499, "Pixel resolution [um/pix]"=w492, "Axes Speeds [mm/s]"=w525, "N pics captured"=3, "Pause before image capture [ms]"=w484, "error in"=w513, "Stage position"=w491, "Record keeping file path"=w512, "Moving"=w493, "XYZ .NET Refnum in"=w487, "Current Build Phase"=w489, "Templates path"=w494, "Current image"=w490, "Calibration Results"=w488) -> ("Cross- check: Are these the center of pins in the center of the image?"=w521:T11[], "Finished!"=w523:bool, "XYZ .NET Refnum out"=w486:refnum<k24>, "Cam session out"=w526:T1, "Angle of pins [rad]"=→"Angle between stave and xyz stage":dbl, "Calibrated stave origin (X,Y) [mm]"=→"Calibrated stave origin (X,Y) [mm]":dbl[], "Calibrated stave basis [mm]"=→"Calibrated stave basis [mm]":dbl[][], "Error report"=w520:errorcluster)  [unwired: 4 in, 1 out]
      n281 = Not(x=w523) -> (.not. x?=w522:bool)
      n282 = call "DumpImageSet (SubVI).vi"("error in (no error)"=w520, "Calibrated Image Array"=w521) -> ("error out"=w503:errorcluster)  [unwired: 6 in]
      n283 = local write "Session Out"(w526) -> ()
      n284 = local write "XYZ Stage Control"(w486) -> ()
      n285 = Merge Errors(w504, w503) -> (w483:errorcluster)
      n286 = local write "Moving"(w522) -> ()
    }
    frame #5 {
      n287 = local write "Calibrated?"(TRUE ("Calibrated?")) -> ()
      n288 = call "LightSwitch (SubVI).vi"() -> ()  [unwired: 12 in]
      n289 = local read "Calibrated module height"() -> (w535:dbl)
      n290 = local write "Current Build Phase"("Fetching the virtual stave..." ("Current Build Phase")) -> ()
      n291 = call "0_PlanVirtualStave.vi"("Working height [mm]"=w535, "N Modules"="N Modules", "Module fiducial marker"="Module fiducial marker", "Tape Type"="Tape Type") -> ("Stave Basis: Coordinates of Fiducials on Modules"=w538:dbl[][])  [unwired: 6 in, 1 out]
    }
    frame #6 {
      n292 = for {
        tunnel: w544 -> [w569] mode=indexing
        tunnel: [w562] -> w543 mode=indexing
        n293 = Index Array(array=w569, index #1=0 ("index"), index #2=1 ("index"), index #3=2 ("index")) -> (element #1=w554:dbl, element #2=w551:dbl, element #3=w555:dbl)
        n294 = local read "Angle between stave and xyz stage"() -> (w566:dbl)
        n295 = local read "Calibrated stave origin (X,Y) [mm]"() -> (w561:dbl[])
        n296 = call "RotateCoordinate (SubVI).vi"("Units"=enum16{"mrad", "Radians", "Degrees"}."Radians", "Angle"=w566, "y"=w551, "x"=w554) -> ("y'"=w552:dbl, "x'"=w553:dbl)  [unwired: 5 in, 1 out]
        n297 = Index Array(array=w561, index #1=0 ("index"), index #2=1 ("index")) -> (element #1=w559:dbl, element #2=w557:dbl)
        n298 = Add(x=w559, y=w553) -> (x+y=w564:dbl)
        n299 = Add(x=w557, y=w552) -> (x+y=w563:dbl)
        n300 = Build Array(w564, w563, w555) -> (w562:dbl[])
      }
      n301 = local read "Tape Type"() -> (w549:enum16{"Stereo", "Axial"})
      n302 = property on="Tape Type" class="Enum (strict)"() -> ("Strings []"=w550:string[])  [unwired: 2 in, 2 out]
      n303 = Index Array(array=w550, index=w549) -> (element=w547:string)
      n304 = Concatenate Strings("Aligning real and virtual " ("Current Build Phase"), w547, " staves..." ("string")) -> (w546:string)
      n305 = local write "Current Build Phase"(w546) -> ()
    }
    frame #7 {
      # "Locking points (based on Sutcliffe drawings), coordinate system reference >>"
      # "Module centres, in the stave basis >>"
      # "Fiducials, in the stave basis >>"
      # "User must confirm coordinates to proceed"
      n306 = local read "Reports path"() -> (w576:path)
      n307 = local read "N Modules"() -> (w579:i32)
      n308 = for {
        N: w579 -> [_]
        tunnel: w577 -> [w607]
        tunnel: [w602] -> w582 mode=indexing
        tunnel: [w601] -> w581 mode=indexing
        i -> [w606]
        w604 = 4 ("x")
        n309 = Multiply(x=w604, y=w606) -> (x*y=w605:i32)
        n310 = Array Subset(array=w607, index (row)=w605, length (row)=w604) -> (w603:dbl[][])  [unwired: 2 in]
        n311 = call "GetModuleCentre (SubVI).vi"("4x3 Array of Fiducial Coordinates"=w603) -> ("x, centre"=w602:dbl, "y, centre"=w601:dbl)
      }
      n312 = Build Path(base path=w576, name or relative path="virtualstave.csv") -> (appended path=w574:path)
      n313 = local read "Calibrated stave basis [mm]"() -> (w583:dbl[][])
      n314 = call-poly <vilib>:"Write Delimited Spreadsheet.vi"("file path (dialog if empty)"=w574, "format (%.3f)"="%.9f", "2D data"=w577, "error in (no error)"=w572, "delimiter (\\t)"="," ("delimiter (\\t)")) -> ("error out"=w570:errorcluster)  [unwired: 9 in, 1 out]
      n315 = Index Array(array=w583, index (col) #1=0 ("disabled index (col)"), index (col) #2=1 ("disabled index (col)")) -> (element #1=w588:dbl[], element #2=w589:dbl[])  [unwired: 2 in]
      n316 = Index Array(array=w577, index (col) #1=0 ("disabled index (col)"), index (col) #2=1 ("index (col)")) -> (element #1=w584:dbl[], element #2=w585:dbl[])  [unwired: 2 in]
      n317 = Bundle("Calibrated stave basis [mm]"=w588, "Calibrated stave basis [mm]"=w589) -> (w593:T19)  [unwired: 1 in]
      n318 = Bundle(w584, w585) -> (w592:cluster{dbl[], dbl[]})  [unwired: 1 in]
      n319 = Bundle(w582, w581) -> (w580:cluster{dbl[], dbl[]})  [unwired: 1 in]
      n320 = local read "Tape Type"() -> (w596:enum16{"Stereo", "Axial"})
      n321 = Build Array(w593, w592, w580) -> (→"Module fiducials in the XYZ stage's basis":T20)
      n322 = property on="Tape Type" class="Enum (strict)"() -> ("Strings []"=w595:string[])  [unwired: 2 in, 2 out]
      n323 = Index Array(array=w595, index=w596) -> (element=w598:string)
      n324 = local write "Current Build Phase"("Positioning modules: Consult VisualizingModulePositions front panel... " ("Current Build Phase")) -> ()
      n325 = Concatenate Strings("Preparing to position modules with " ("Current Build Phase"), w598, " stave coordinates..." ("string")) -> (w599:string)
      n326 = local write "Current Build Phase"(w599) -> ()
    }
    frame #8 {
      n327 = disable-structure shown="Disabled" {
        frame Disabled {
          # "PER MODULE"
          n328 = for {
            N: 13 -> [_]
            i -> [w627]
            n329 = flat-sequence {
              tunnel: w627 -> [w628]
              tunnel: w627 -> [w635]
              frame #0 {
                n330 = Number To Decimal String(number=w628) -> (decimal integer string=w630:string)  [unwired: 1 in]
                n331 = Concatenate Strings("Applying glue for module #" ("Current Build Phase"), w630, "..." ("string")) -> (w632:string)
                n332 = local write "Current Build Phase"(w632) -> ()
              }
              frame #1 {
                n333 = Number To Decimal String(number=w635) -> (decimal integer string=w636:string)  [unwired: 1 in]
                n334 = Concatenate Strings("Positioning module #" ("Current Build Phase"), w636, "..." ("string")) -> (w633:string)
                n335 = local write "Current Build Phase"(w633) -> ()
              }
            }
          }
        }
        frame Enabled {
        }
      }
      n336 = control-ref of="Current stage position [mm]"() -> (w617:refnum<vi>)
      n337 = local read "Module fiducial marker"() -> (w615:T9)
      n338 = control-ref of="Module Progress Report"() -> (w619:refnum<vi>)
      n339 = local read "Average microns/pixel"() -> (w613:ext)
      n340 = local read "XYZ Stage Control"() -> (w609:refnum<k24>)
      n341 = control-ref of="Current field of view"() -> (w618:refnum<vi>)
      n342 = control-ref of="Current Build Phase"() -> (w611:refnum<vi>)
      n343 = local read "Session Out"() -> (w625:T1)
      n344 = local read "Axis Speeds"() -> (w612:T10)
      n345 = local read "N Modules"() -> (w622:i32)
      n346 = local read "Code path"() -> (w621:path)
      n347 = control-ref of="Moving"() -> (w616:refnum<vi>)
      n348 = call "2_VisualizeModulePositioning.vi"("Session in"=w625, "Calibrated positions of fiducials [mm]"=w623, "XYZ .NET Refnum in"=w609, "Axis Speeds"=w612, "Module fiducial marker"=w615, "N modules"=w622, "error in (no error)"=w608, "Templates path"=w621, "Calibration [um/pix]"=w613, "Current Build Phase"=w611, "Placement tolerance [um]"="Placement tolerance [um]", "Current Image"=w618, "Current stage position"=w617, "Module Report"=w619, "Moving"=w616) -> ("Session Out"=w624:T1, "XYZ .NET Refnum out"=w610:refnum<k24>, "error out"=w620:errorcluster)  [unwired: 10 in]
      n349 = local write "Session Out"(w624) -> ()
      n350 = local write "Program Errors"(w620) -> ()
      n351 = local write "XYZ Stage Control"(w610) -> ()
    }
    frame #9 {
      n352 = local read "Tape Type"() -> (w642:enum16{"Stereo", "Axial"})
      n353 = local write "Mounted?"(TRUE ("Calibrated?")) -> ()
      n354 = property on="Tape Type" class="Enum (strict)"() -> ("Strings []"=w641:string[])  [unwired: 2 in, 2 out]
      n355 = Index Array(array=w641, index=w642) -> (element=w640:string)
      n356 = Concatenate Strings(w640, " stave side complete! " ("Current Build Phase")) -> (w643:string)
      n357 = local write "Current Build Phase"(w643) -> ()
    }
    frame #10 {
      # "import contents of visually inspect list of coordinates\nso that they display on the front panel"
      n358 = local read "Tape Type"() -> (w645:enum16{"Stereo", "Axial"})
      n359 = property on="Tape Type" class="Enum (strict)"() -> ("Strings []"=w646:string[])  [unwired: 2 in, 2 out]
      n360 = Index Array(array=w646, index=w645) -> (element=w647:string)
      n361 = Concatenate Strings(w647, " stave side survey in progress... " ("Current Build Phase")) -> (w644:string)
      n362 = local write "Current Build Phase"(w644) -> ()
    }
    frame #11 {
      n363 = local read "Session Out"() -> (w649:T1)
      n364 = local read "Tape Type"() -> (w654:enum16{"Stereo", "Axial"})
      n365 = local write "Surveyed?"(TRUE ("Calibrated?")) -> ()
      n366 = property on="Tape Type" class="Enum (strict)"() -> ("Strings []"=w653:string[])  [unwired: 2 in, 2 out]
      n367 = call <vilib>:"IMAQdx Close Camera.vi"("Session In"=w649) -> ()  [unwired: 10 in, 1 out]
      n368 = Index Array(array=w653, index=w654) -> (element=w652:string)
      n369 = Concatenate Strings(w652, " stave side complete! " ("Current Build Phase")) -> (w655:string)
      n370 = local write "Current Build Phase"(w655) -> ()
    }
  }
